vi "Randomize.vi"(11 "Quantity":T2={"Name"="newQ", "Value"=[], "Uncertainty"=[], "Degrees of\nFreedom"=[], "Correlation"=[], "Randomized uncertainty"=[]}) -> ()   [LabVIEW 2013]
uses:
  qwtblvlib/TD Quantity.ctl
  <vilib>/gmath/statdist.llb/Normal Random.vi
  <vilib>/gmath/statdist.llb/Uniform Random.vi
  <vilib>/gmath/statdist.llb/Student t Random.vi
  <vilib>/gmath/NI_Gmath.lvlib
  <vilib>/Analysis/NI_AALBase.lvlib
  qwtblvlib/QWTBLVLib.lvlib
panel:
  out "Randomization for quantity:":string
  in  "xmax":dbl=1.0
  in  "xmin":dbl
  in  "Distribution type":T1(ring)
  in  "k degrees of freedom":i32=1
  in  "mean":dbl
  in  "std":dbl=1.0
  in  "Seed":i32=-1
  in  "Cancel Button":bool
  in  "OK Button":bool
  out "Histogram Graph":T3(graph)
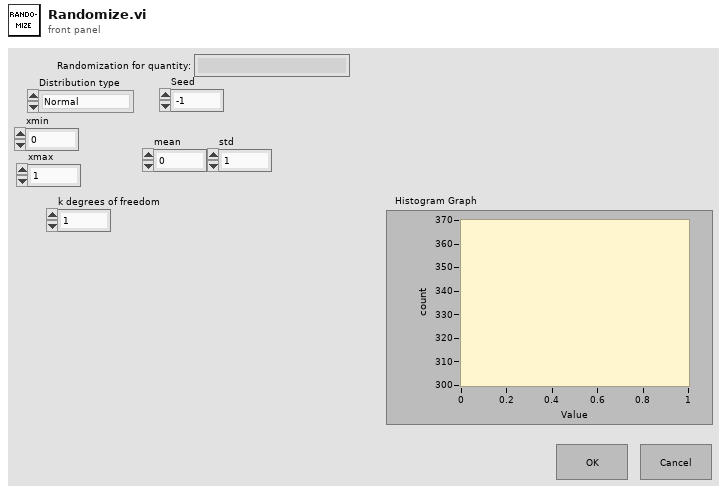
[diagram p1: front panel]
types:
  T1 = enum32{"Normal", "Student t", "Triangular", "Uniform"}
  T2 = typedef "QWTBLVLib.lvlib/TD Quantity.ctl" = cluster{"Name":string, "Value":dbl[][], "Uncertainty":dbl[][], "Degrees of\nFreedom":dbl[][], "Correlation":dbl[][], "Randomized uncertainty":dbl[][]}
  T3 = cluster{"X Values":dbl[], "Histogram: h(x)":i32[]}
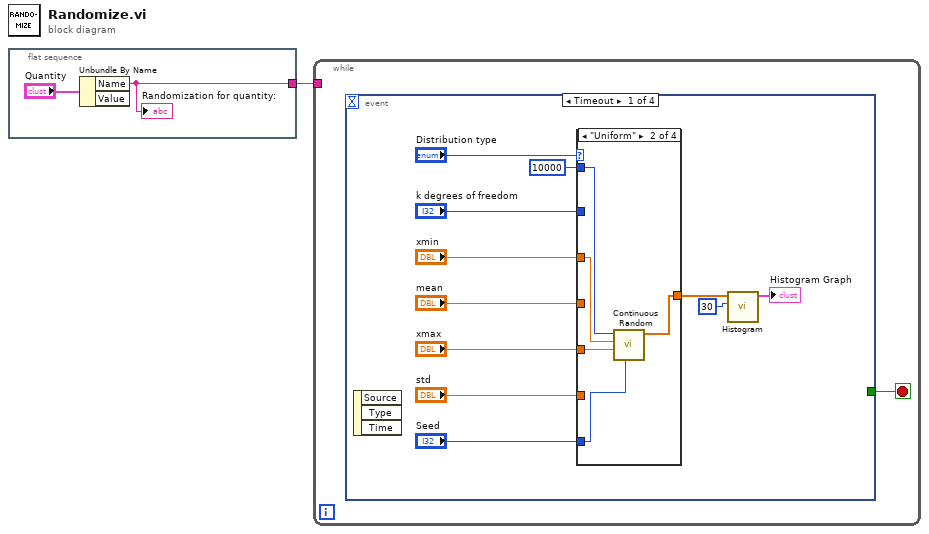
[diagram p0: block diagram]
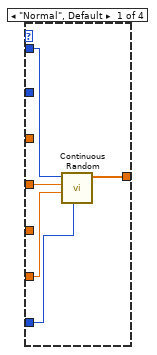
[diagram p2: hidden frame]
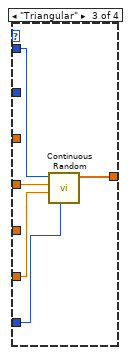
[diagram p3: hidden frame]
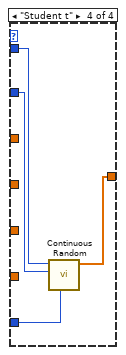
[diagram p4: hidden frame]
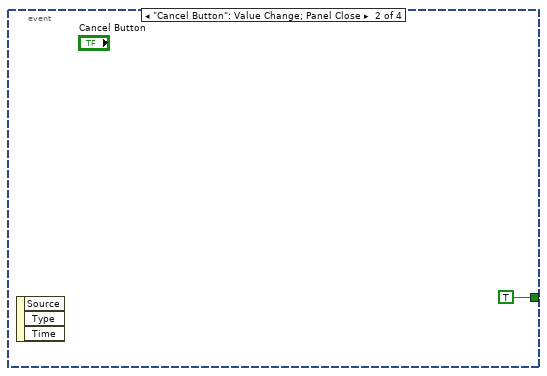
[diagram p5: hidden frame]
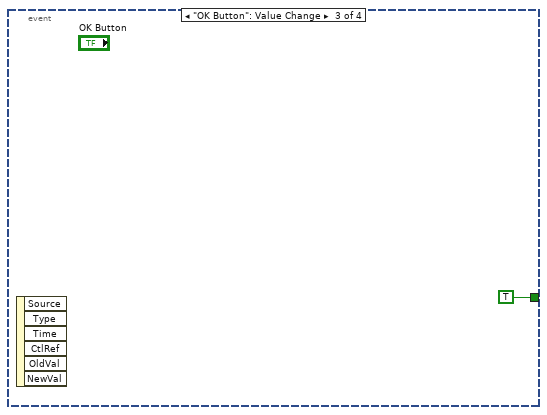
[diagram p6: hidden frame]
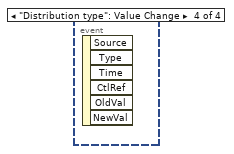
[diagram p7: hidden frame]
diagram:
  n1 = flat-sequence {
    tunnel: [w2] -> w1
    frame #0 {
      n2 = Unbundle By Name("Quantity") -> ("Name"=w2:string)  [unwired: 1 out]
      "Randomization for quantity:" <- w2
    }
  }
  n3 = while {
    tunnel: w1 -> [_]
    stop <- w4 stop-if-true
    n4 = event shown="[0] Timeout" {
      selector: _ -> [_ _ _ _]
      dyn-events: _ -> [_ _ _ _]
      timeout: _ -> [_ _ _ _]
      tunnel: [_ TRUE TRUE _] -> w4
      event Timeout {
        n5 = event-data() -> ()  [unwired: 1 in, 3 out]
        n6 = case shown="\"Uniform\"" "Distribution type" {
          tunnel: [w20 w24 w27 w34] -> w15
          tunnel: 10000 ("samples") -> [w19 w25 w26 w33]
          tunnel: "k degrees of freedom" -> [_ _ _ w32]
          tunnel: "mean" -> [w18 _ w30 _]
          tunnel: "std" -> [w17 _ w29 _]
          tunnel: "Seed" -> [w16 w23 w28 w31]
          tunnel: "xmax" -> [_ w22 _ _]
          tunnel: "xmin" -> [_ w21 _ _]
          frame "Normal", Default {
            n7 = call-poly <vilib>:"Continuous Random.vi"("seed"=w16, "std"=w17, "mean"=w18, "samples"=w19) -> ("normal random data"=w20:dbl[])  [unwired: 6 in, 1 out]
          }
          frame "Uniform" {
            n8 = call-poly <vilib>:"Continuous Random.vi"("seed"=w23, "xmax"=w22, "xmin"=w21, "samples"=w25) -> ("uniform random data"=w24:dbl[])  [unwired: 6 in, 1 out]
          }
          frame "Triangular" {
            n9 = call-poly <vilib>:"Continuous Random.vi"("seed"=w28, "std"=w29, "mean"=w30, "samples"=w26) -> ("normal random data"=w27:dbl[])  [unwired: 6 in, 1 out]
          }
          frame "Student t" {
            n10 = call-poly <vilib>:"Continuous Random.vi"("seed"=w31, "k degrees of freedom"=w32, "samples"=w33) -> ("Student t random data"=w34:dbl[])  [unwired: 7 in, 1 out]
          }
        }
        n11 = call <vilib>:"Histogram.vi"("intervals"=30, "X"=w15) -> ("Histogram Graph"=→"Histogram Graph":T3)  [unwired: 6 in, 3 out]
      }
      event "Cancel Button": Value Change; Panel Close {
        n12 = event-data() -> ()  [unwired: 1 in, 3 out]
      }
      event "OK Button": Value Change {
        n13 = event-data() -> ()  [unwired: 1 in, 6 out]
      }
      event "Distribution type": Value Change {
        n14 = event-data() -> ()  [unwired: 1 in, 6 out]
      }
    }
  }
